vi "write cache to binary.vi"(8 "error in":errorcluster, 10 "cache in":T1, 11 "bin file in":refnum<file>) -> (0 "error out":errorcluster, 2 "cache out":T1, 3 "bin file out":refnum<file>)   [LabVIEW 2013, in "Binary datalogger runtime.lvclass"]
uses:
  Binary datalogger runtime.lvclass
  data cache.ctl
  <vilib>/NI/Tag Bus/table/data table.ctl
  <vilib>/NI/Tag Bus/table/data table.lvlib
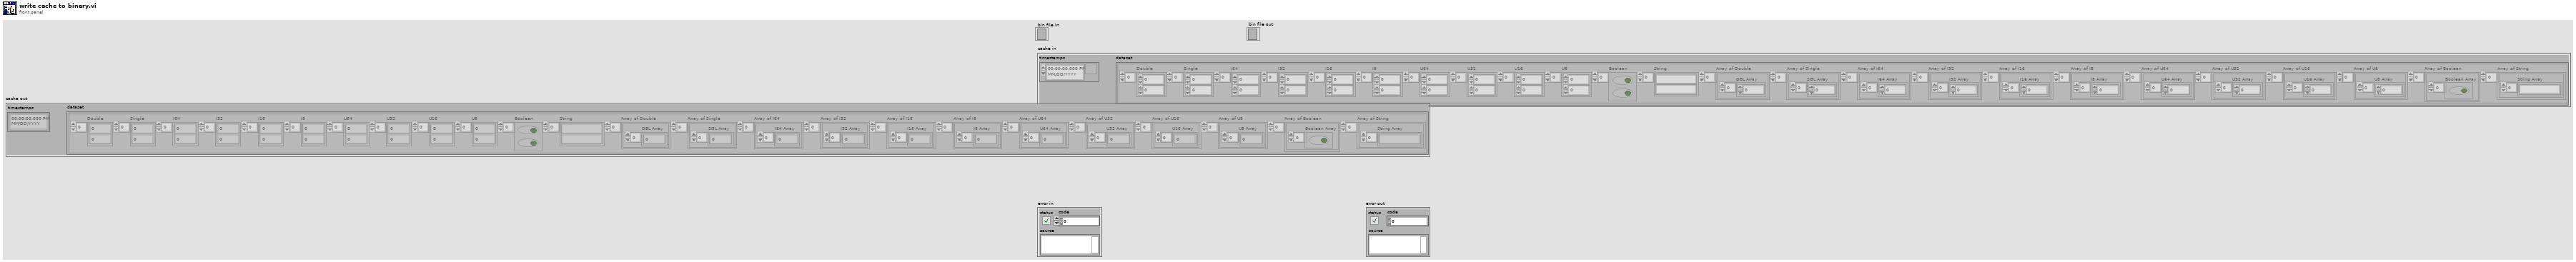
[diagram p1: front panel]
types:
  T1 = typedef "Binary datalogger runtime.lvclass/data cache.ctl" = cluster{"timestamps":timestamp[], "dataset":T2[]}
  T2 = typedef "tag bus.lvlib/data table.lvlib/data table.ctl" = cluster{"Double":dbl[], "Single":sgl[], "I64":i64[], "I32":i32[], "I16":i16[], "I8":i8[], "U64":u64[], "U32":u32[], "U16":u16[], "U8":u8[], "Boolean":bool[], "String":string[], "Array of Double":cluster{"DBL Array":dbl[]}[], "Array of Single":cluster{"SGL Array":sgl[]}[], "Array of I64":cluster{"I64 Array":i64[]}[], "Array of I32":cluster{"I32 Array":i32[]}[], "Array of I16":cluster{"I16 Array":i16[]}[], "Array of I8":cluster{"I8 Array":i8[]}[], "Array of U64":cluster{"U64 Array":u64[]}[], "Array of U32":cluster{"U32 Array":u32[]}[], "Array of U16":cluster{"U16 Array":u16[]}[], "Array of U8":cluster{"U8 Array":u8[]}[], "Array of Boolean":cluster{"Boolean Array":bool[]}[], "Array of String":cluster{"String Array":string[]}[]}
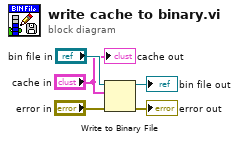
[diagram p0: block diagram]
diagram:
  n1 = Write to Binary File(file (use dialog)="bin file in", data="cache in", error in="error in") -> (refnum out=→"bin file out":refnum<file>, error out=→"error out":errorcluster)  [unwired: 3 in, 1 out]
  "cache out" <- "cache in"
